vi "Protocol Write.vi"(8 "error in (no error)":errorcluster, 9 "timeout":i32=10000, 10 "data":u8[](array[numeric]), 11 "protocol layer in":refnum<class "Serial Slave.lvclass">) -> (0 "error out":errorcluster, 1 "timed out?":bool, 3 "protocol layer out":refnum<class "Serial Slave.lvclass">)   [LabVIEW 2020, in "SubVIs.lvlib" / "Serial Slave.lvclass"]
doc: "This provides an interface for writing to a network bus."
uses:
  <vilib>/Modbus/subvis/Protocol/Serial/Serial Slave/Serial Slave.lvclass
  <vilib>/Modbus/subvis/Protocol/Serial/Serial Slave/Serial Slave.lvclass/Serial Slave.ctl
  <vilib>/Modbus/subvis/Protocol/Serial/Serial Shared Components/Serial Shared Components.lvlib
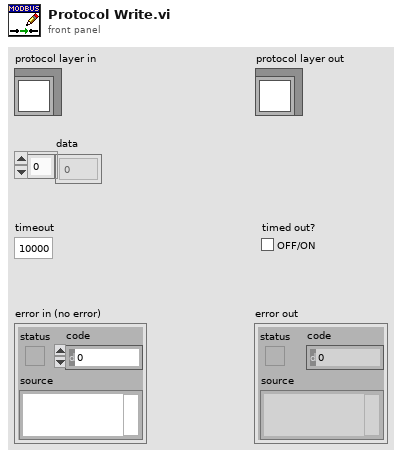
[diagram p1: front panel]
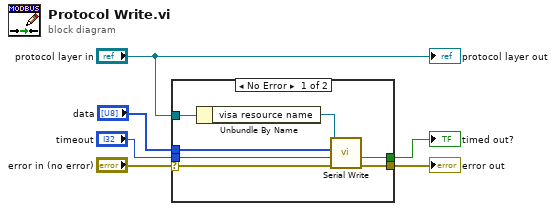
[diagram p0: block diagram]
diagram:
  n1 = case shown="No Error" "error in (no error)" {
    selector: "error in (no error)" -> [w7 w14]
    tunnel: "timeout" -> [w12 _]
    tunnel: "data" -> [w11 _]
    tunnel: "protocol layer in" -> [w10 _]
    tunnel: [w9 w14] -> w3
    tunnel: [w8 _] -> w2
    frame No Error {
      n2 = Unbundle By Name(w10) -> ("visa resource name"=w13:refnum<visa-resource-name>)
      n3 = call <vilib>:"Serial Write.vi"("error in (no error)"=w7, "timeout (ms)"=w12, "data"=w11, "VISA resource"=w13) -> ("error out"=w9:errorcluster, "timed out?"=w8:bool)  [unwired: 6 in]
    }
    frame Error {
    }
  }
  "error out" <- w3
  "timed out?" <- w2
  "protocol layer out" <- "protocol layer in"
